vi "修改累积剂量报警阈值.vi"(8 "待修改探头":string[](array[string]), 11 "累积剂量 i":T1(array[cluster])) -> (3 "累积剂量 o":T1(array[cluster]))   [LabVIEW 2017]
uses:
  <vilib>/Utility/xml.llb/Write to XML File(string).vi
panel:
  in  "取消":bool
  in  "确定":bool
  in  "累积阈值":dbl=1000.0
  in  "单位":enum8{"μSv", "mSv"}(ring)
  # "累积报警阈值"
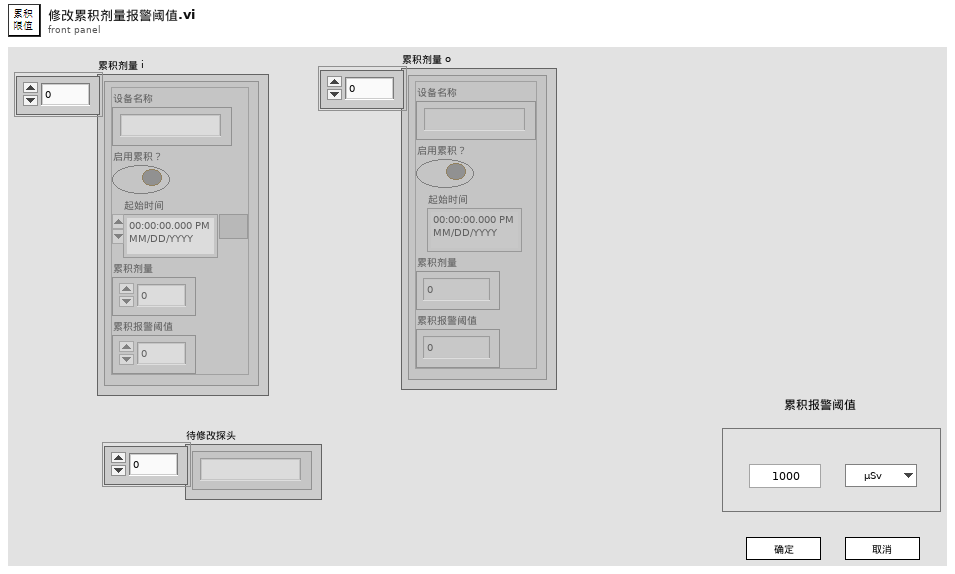
[diagram p1: front panel]
types:
  T1 = cluster{"设备名称":string, "启用累积？":bool, "起始时间":timestamp, "累积剂量":dbl, "累积报警阈值":dbl}[]
  T2 = enum32{"Invalid", "Standard", "Closed", "Hidden", "Minimized", "Maximized"}
  T3 = cluster{"设备名称":string, "启用累积？":bool, "起始时间":timestamp, "累积剂量":dbl, "累积报警阈值":dbl}
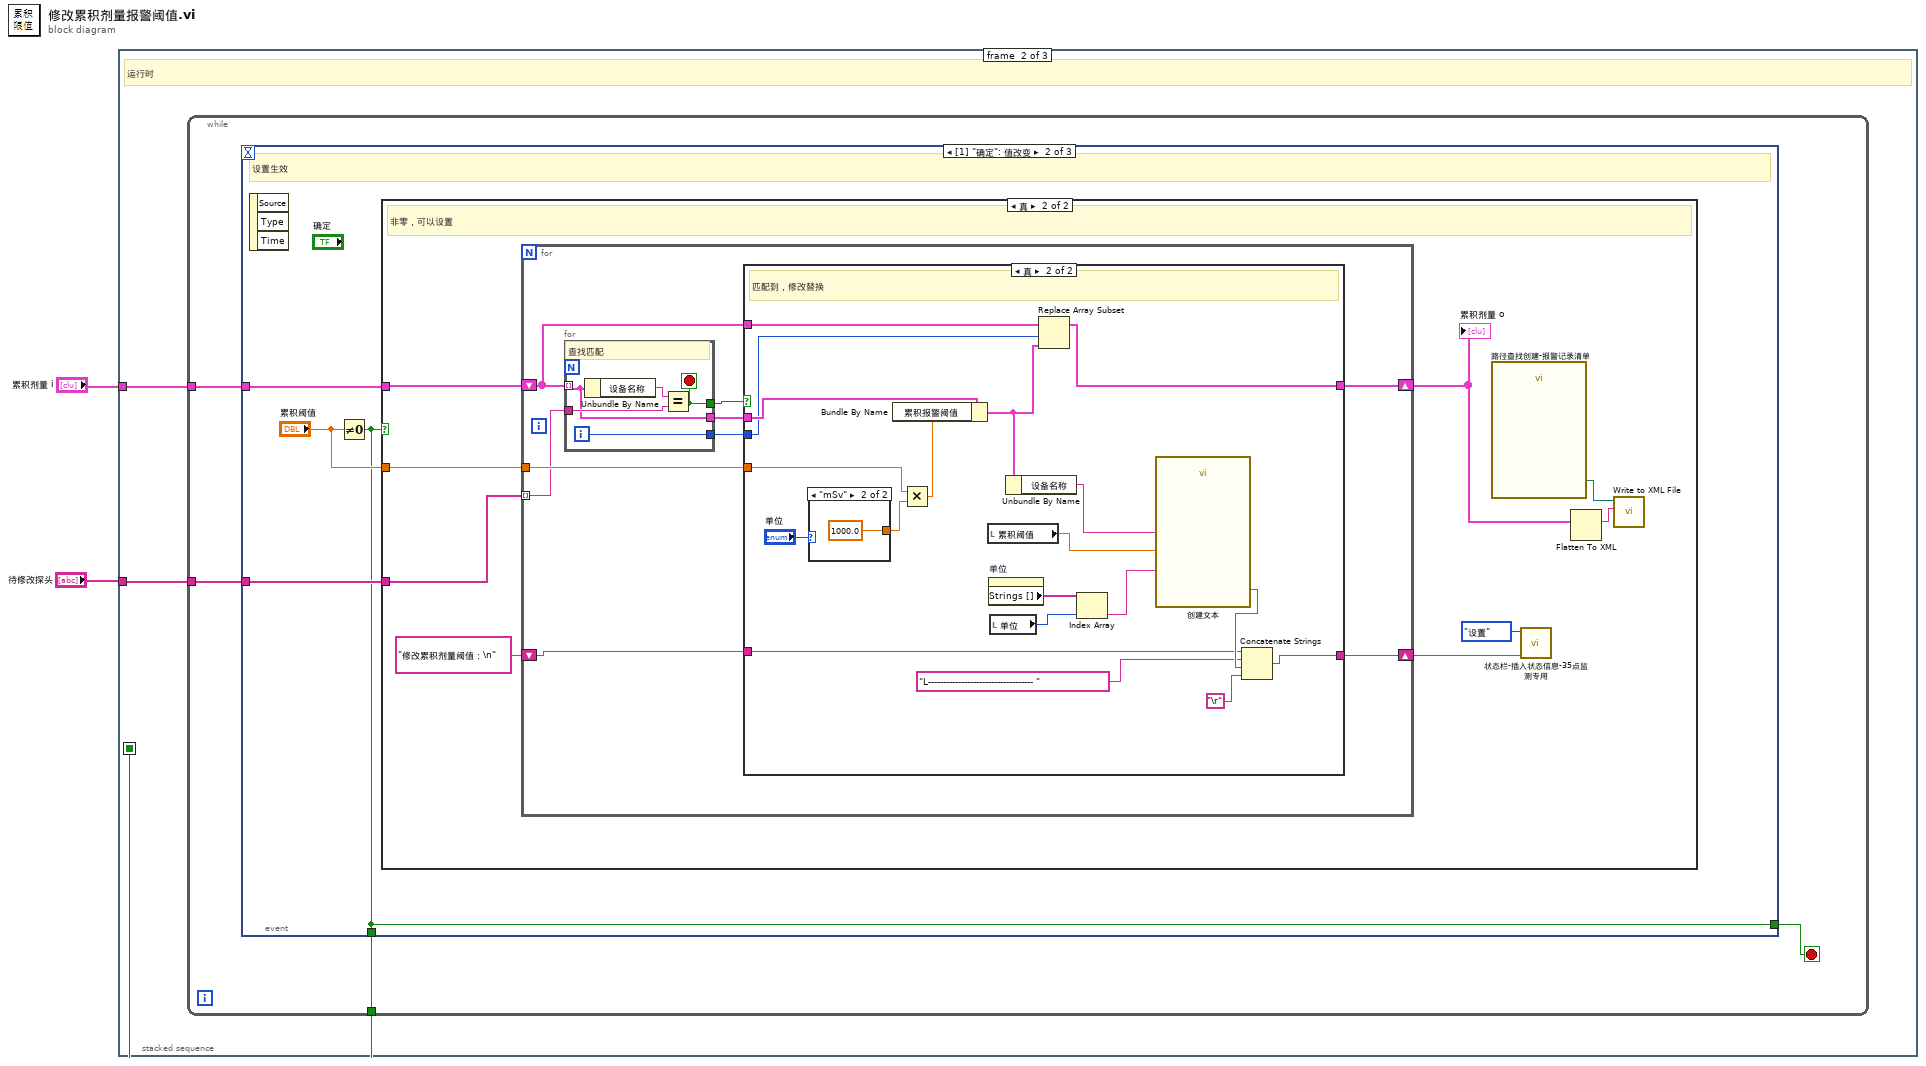
[diagram p0: block diagram]
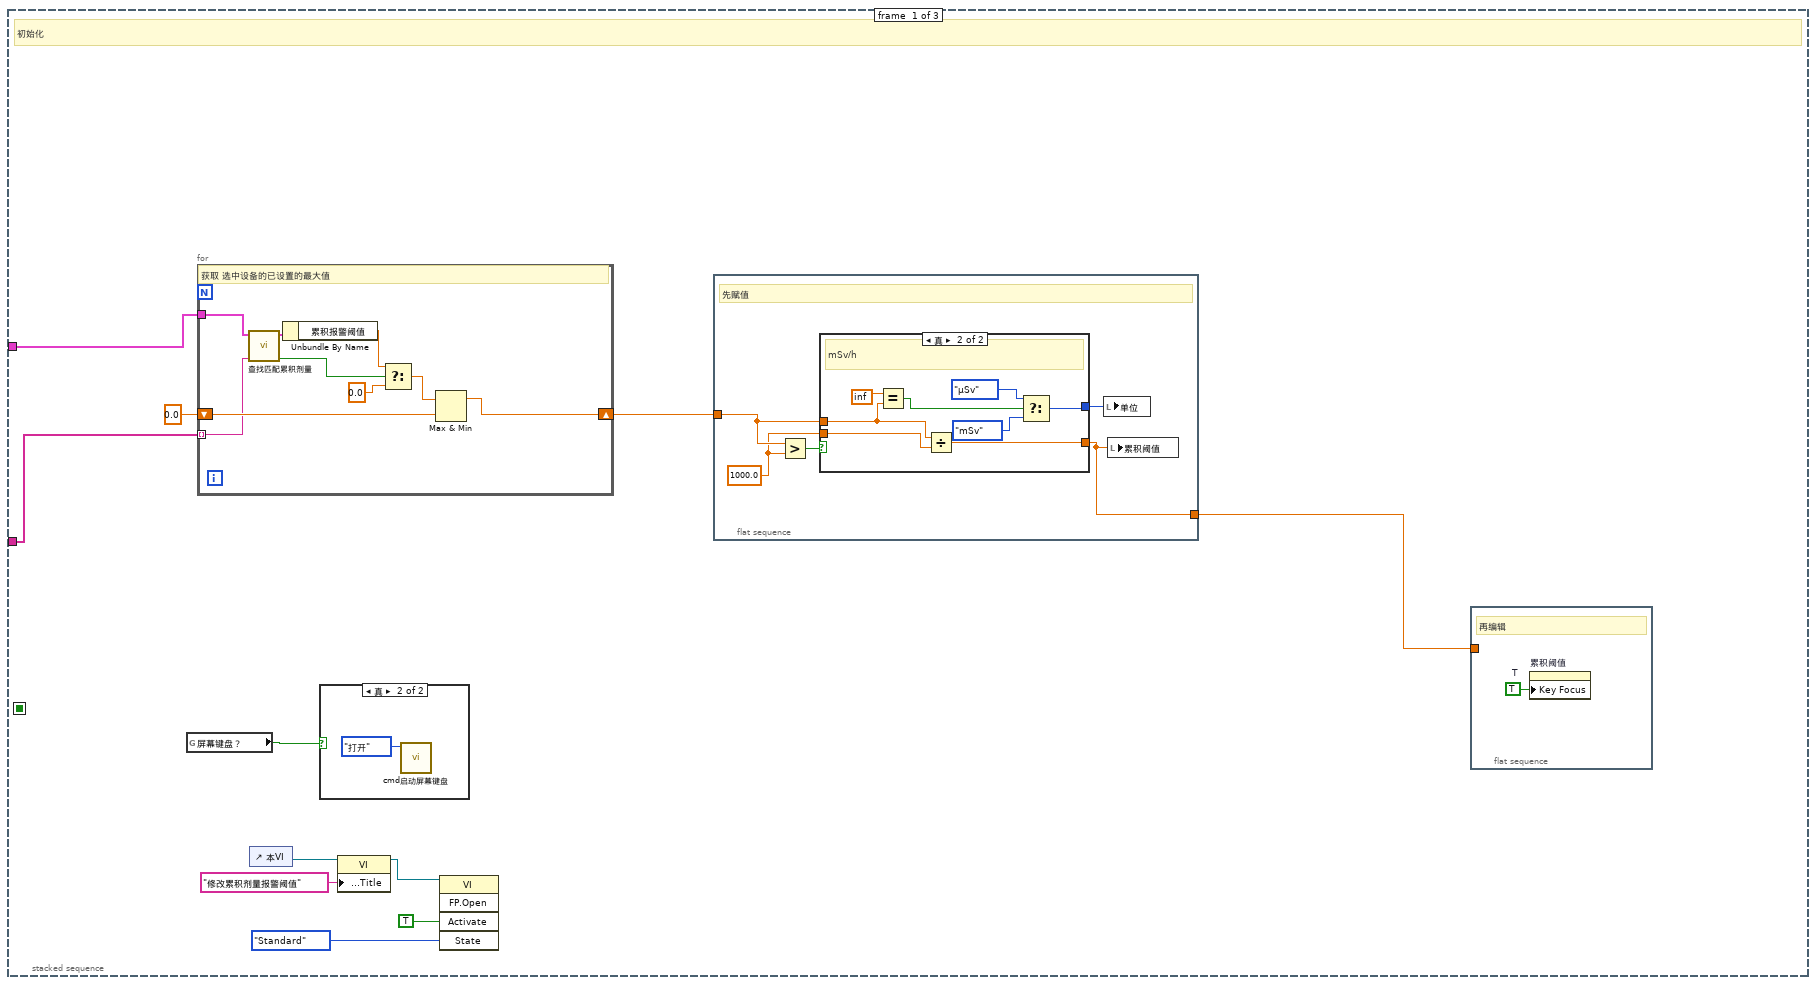
[diagram p2: hidden frame]
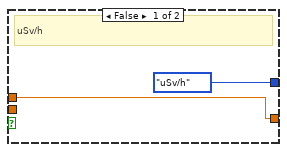
[diagram p3: hidden frame]
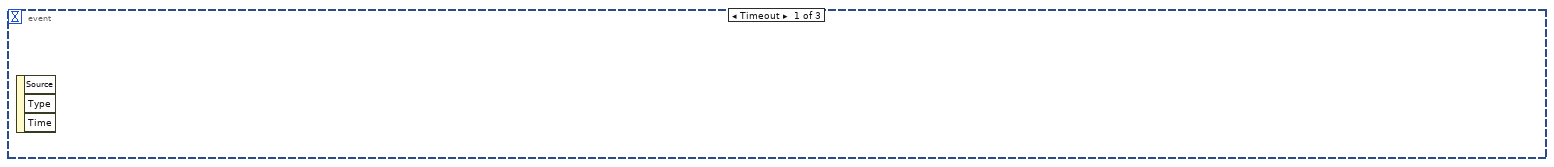
[diagram p5: hidden frame]
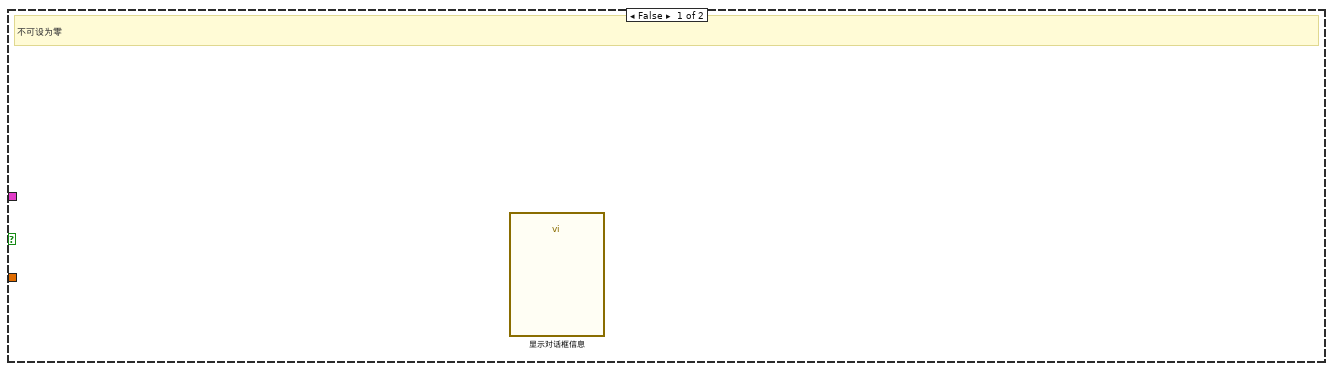
[diagram p6: hidden frame]
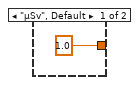
[diagram p8: hidden frame]
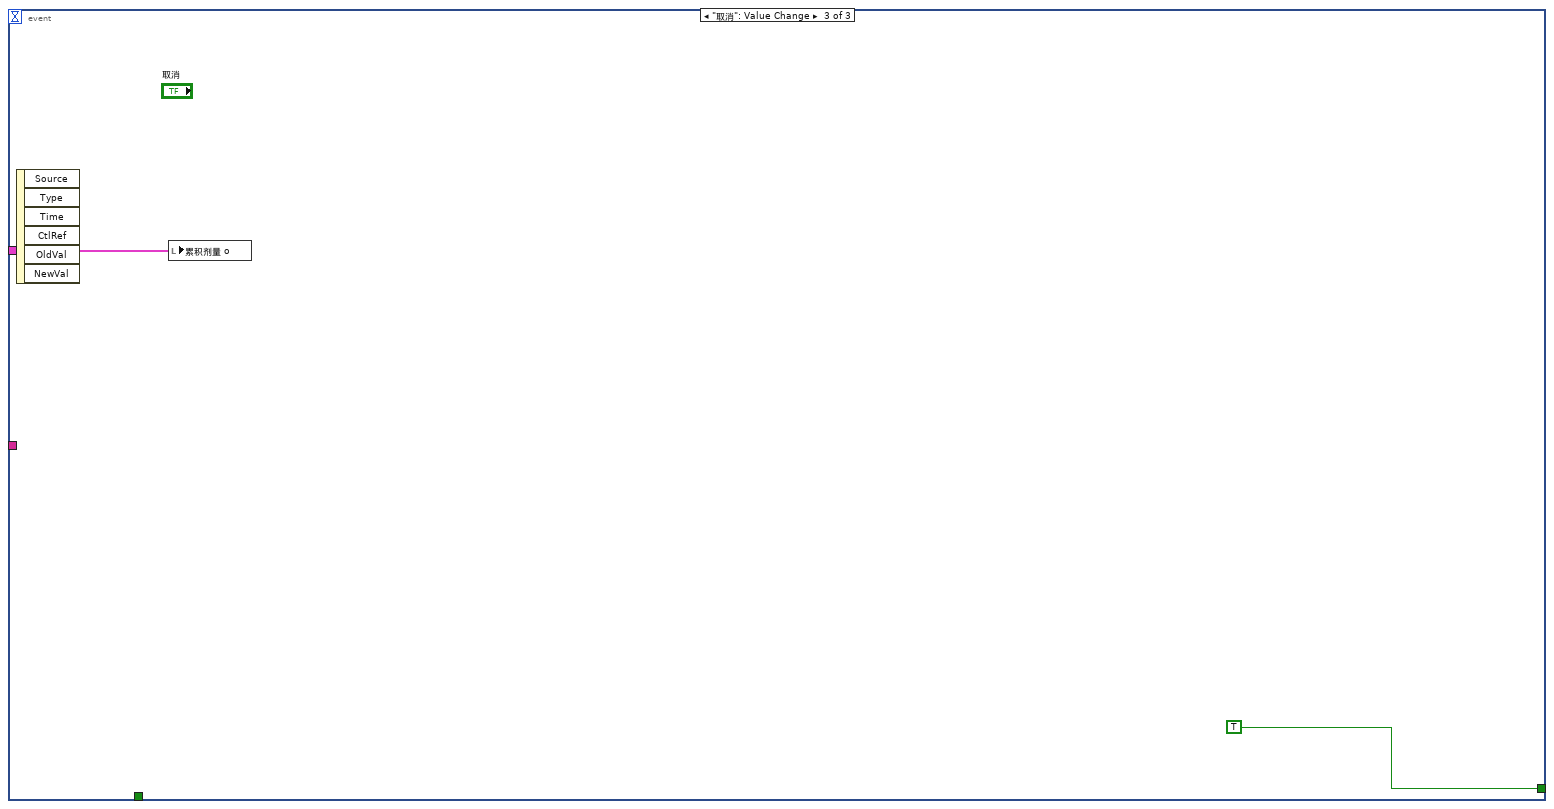
[diagram p9: hidden frame]
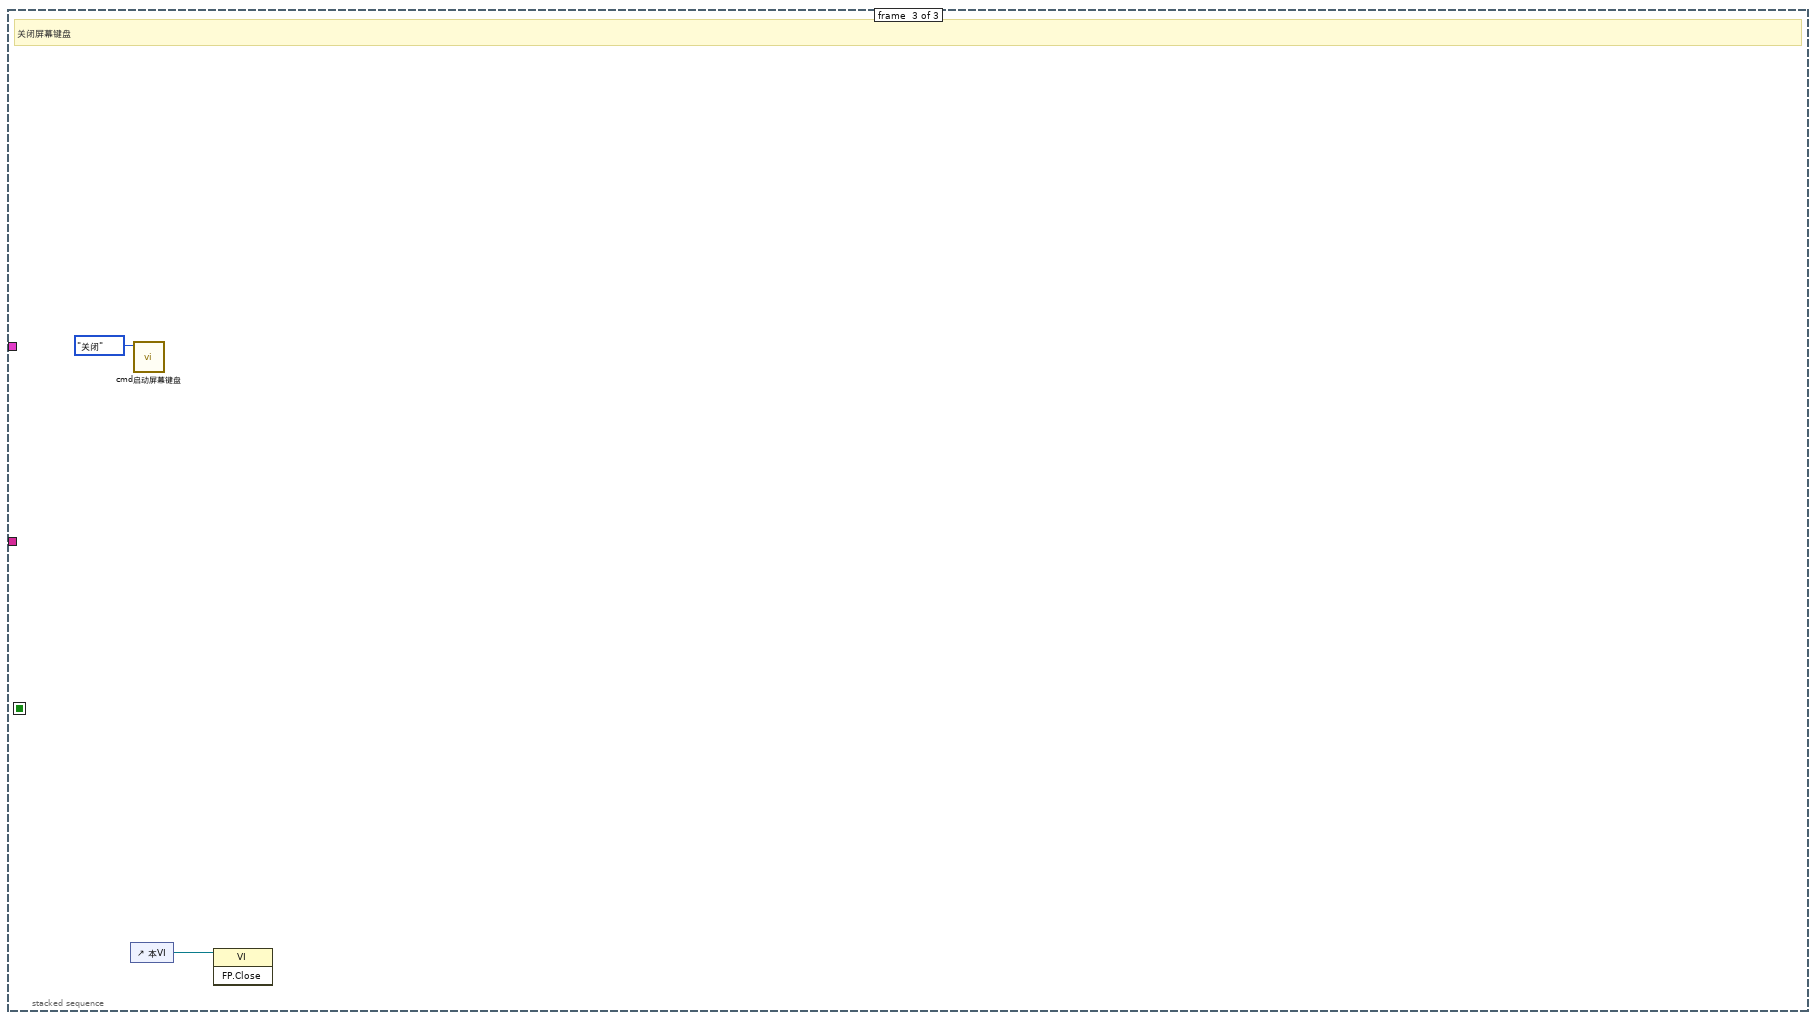
[diagram p10: hidden frame]
diagram:
  n1 = stacked-sequence {
    seq-local: [_ w40 _] -> [_ _ _]
    tunnel: "累积剂量 i" -> [w12 w41 _]
    tunnel: "待修改探头" -> [w11 w42 _]
    frame #0 {
      # "初始化"
      n2 = global read "全局变量-35点监测.vi" "屏幕键盘？"() -> (w9:bool)
      n3 = for {
        tunnel: w11 -> [w36] mode=indexing
        shift-right: [w38] -> w10
        shift-left: 0.0 ("累积剂量") -> [w39]
        tunnel: w12 -> [w37]
        # "获取 选中设备的已设置的最大值"
        n4 = call "查找匹配累积剂量.vi"("探头名称"=w36, "累积剂量"=w37) -> ("匹配？"=w35:bool, "匹配的累积剂量"=w34:T3)  [unwired: 7 in, 1 out]
        n5 = Unbundle By Name(w34) -> ("累积报警阈值"=w33:dbl)
        n6 = Select(t=w33, s=w35, f=0.0 ("累积剂量")) -> (s? t:f=w31:dbl)
        n7 = Max & Min ("最大值与最小值")(x=w31, y=w39) -> (max(x,y)=w38:dbl)  [unwired: 1 out]
      }
      n8 = control-ref of="本VI"() -> (w7:refnum<vi>)
      n9 = case shown="真" w9 {
        frame False {
        }
        frame True {
          n10 = call "cmd启动屏幕键盘.vi"("软键盘开关"=enum16{"关闭", "打开"}."打开") -> ()  [unwired: 9 in, 2 out]
        }
      }
      n11 = property class="VI"(reference=w7, "Front Panel.Title"="修改累积剂量报警阈值" ("前面板窗口:标题")) -> (reference out=w4:refnum<vi>)  [unwired: 1 in, 1 out]
      n12 = invoke class="VI" method="FP.Open"(reference=w4, "Activate"=TRUE ("激活？"), "State"=T2."Standard" ("状态")) -> ()  [unwired: 2 in, 5 out]
      n13 = flat-sequence {
        tunnel: w10 -> [w17]
        tunnel: [w14] -> w3
        frame #0 {
          w16 = 1000.0 ("y")
          # "先赋值"
          n14 = Greater?(x=w17, y=w16) -> (0:w18:bool)
          n15 = case shown="真" w18 {
            tunnel: w17 -> [w19 w26]
            tunnel: w16 -> [_ w28]
            tunnel: [w19 w27] -> w14
            tunnel: [enum8{"uSv/h", "mSv/h"}."uSv/h" ("单位1") w22] -> w15
            frame False {
              # "uSv/h"
            }
            frame True {
              # "mSv/h"
              n16 = Equal?(x=inf, y=w26) -> (x = y?=w24:bool)
              n17 = Divide(x=w26, y=w28) -> (x/y=w27:dbl)
              n18 = Select(t=enum8{"μSv", "mSv"}."μSv" ("单位1"), s=w24, f=enum8{"μSv", "mSv"}."mSv" ("单位1")) -> (s? t:f=w22:enum8{"μSv", "mSv"})
            }
          }
          n19 = local write "单位"(w15) -> ()
          n20 = local write "累积阈值"(w14) -> ()
        }
      }
      n21 = flat-sequence {
        tunnel: w3 -> [_]
        frame #0 {
          w29 = TRUE  # T
          # "再编辑"
          n22 = property on="累积阈值" class="DigNum (严格)"("Key Focus"=w29) -> ()  [unwired: 2 in, 2 out]
        }
      }
    }
    frame #1 {
      # "运行时"
      n23 = while {
        tunnel: w42 -> [w46]
        tunnel: w41 -> [w45]
        tunnel: [w43] -> w40
        stop <- w44 stop-if-true
        n24 = event shown="[1] \"确定\": 值改变" {
          selector: _ -> [_ _ _]
          dyn-events: _ -> [_ _ _]
          timeout: _ -> [_ _ _]
          tunnel: w46 -> [_ w50 _]
          tunnel: w45 -> [_ w49 w97]
          tunnel: [_ w47 TRUE] -> w44
          tunnel: [_ w47 _] -> w43
          event Timeout {
            n25 = event-data() -> ()  [unwired: 1 in, 3 out]
          }
          event "确定": Value Change {
            # "设置生效"
            n26 = event-data() -> ()  [unwired: 1 in, 3 out]
            n27 = Not Equal To 0?(x="累积阈值") -> (x != 0?=w47:bool)
            n28 = case shown="真" w47 {
              tunnel: w50 -> [_ w58]
              tunnel: w49 -> [_ w59]
              tunnel: "累积阈值" -> [_ w57]
              frame False {
                # "不可设为零"
                n29 = call "显示对话框信息"() -> ()  [unwired: 10 in, 2 out]
              }
              frame True {
                # "非零，可以设置"
                n30 = for {
                  tunnel: w58 -> [w67] mode=indexing
                  tunnel: w57 -> [w68]
                  shift-right: [w60] -> w54
                  shift-left: "修改累积剂量阈值：\n" -> [w61]
                  shift-right: [w62] -> w51
                  shift-left: w59 -> [w65]
                  n31 = for {
                    tunnel: w65 -> [w69] mode=indexing
                    tunnel: w67 -> [w72]
                    tunnel: [w71] -> w64
                    tunnel: [w70] -> w66
                    tunnel: [w69] -> w63
                    i -> [w71]
                    stop <- w70 stop-if-true
                    # "查找匹配"
                    n32 = Unbundle By Name(w69) -> ("设备名称"=w73:string)
                    n33 = Equal?(x=w73, y=w72) -> (x = y?=w70:bool)
                  }
                  n34 = case shown="真" w66 {
                    tunnel: w65 -> [w75 w90]
                    tunnel: [w75 w87] -> w62
                    tunnel: w68 -> [_ w92]
                    tunnel: w64 -> [_ w88]
                    tunnel: w63 -> [_ w89]
                    tunnel: w61 -> [w74 w77]
                    tunnel: [w74 w76] -> w60
                    frame False {
                      # "未匹配，不清零"
                    }
                    frame True {
                      # "匹配到，修改替换"
                      n35 = case shown="\"mSv\"" "单位" {
                        tunnel: [sgl 1.0 ("探头报警值") sgl 1000.0 ("探头报警值")] -> w93
                        frame "μSv", Default {
                        }
                        frame "mSv" {
                        }
                      }
                      n36 = Multiply(x=w92, y=w93) -> (x*y=w91:dbl)
                      n37 = Bundle By Name(cluster=w89, "累积报警阈值"=w91) -> (w79:T3)
                      n38 = local read "累积阈值"() -> (w83:dbl)
                      n39 = property on="单位" class="Enum (严格)"() -> ("Strings []"=w84:string[])  [unwired: 2 in, 2 out]
                      n40 = local read "单位"() -> (w85:enum8{"μSv", "mSv"})
                      n41 = Unbundle By Name(w79) -> ("设备名称"=w78:string)
                      n42 = Replace Array Subset(array=w90, new element=w79, index=w88) -> (w87:T1)
                      n43 = Index Array(array=w84, index=w85) -> (element=w86:string)
                      n44 = call "创建文本"("名称"=w78, "数值"=w83, "单位"=w86) -> ("Result"=w82:string)  [unwired: 11 in, 1 out]
                      n45 = Concatenate Strings(w77, "L----------------------------------- " ("字符串"), w82, "\r") -> (w76:string)
                    }
                  }
                }
                "累积剂量 o" <- w51
                n46 = call "路径查找创建-报警记录清单.vi"() -> ("累积剂量配置文件"=w52:path)  [unwired: 8 in, 11 out]
                n47 = call "状态栏-插入状态信息-35点监测专用.vi"("消息内容"=w54, "状态类型"=enum16{"全部", "报警", "通信", "设置"}."设置") -> ()  [unwired: 10 in]
                n48 = Flatten To XML(anything=w51) -> (xml string=w53:string)
                n49 = call-poly <vilib>:"Write to XML File.vi"("XML Input"=w53, "XML File Path"=w52) -> ()  [unwired: 7 in, 3 out]
              }
            }
          }
          event "取消": Value Change {
            n50 = event-data() -> ()  [unwired: 1 in, 6 out]
            n51 = local write "累积剂量 o"(w97) -> ()
          }
        }
      }
    }
    frame #2 {
      # "关闭屏幕键盘"
      n52 = control-ref of="本VI"() -> (w99:refnum<vi>)
      n53 = call "cmd启动屏幕键盘.vi"("软键盘开关"=enum16{"关闭", "打开"}."关闭") -> ()  [unwired: 9 in, 2 out]
      n54 = invoke class="VI" method="FP.Close"(reference=w99) -> ()  [unwired: 2 in, 3 out]
    }
  }
